vi "timestamp_to_postgres_date.vi"(8 "error in (no error)":errorcluster, 10 "utc":bool, 11 "date_time":dbl format="%^<%H:%M:%S%4u %m/%d/%y>T") -> (0 "error out":errorcluster, 3 "postgres_date":string)   [LabVIEW 2015, in "lv-example-postgres.lvlib"]
uses:
  lv-example-postgres.lvlib
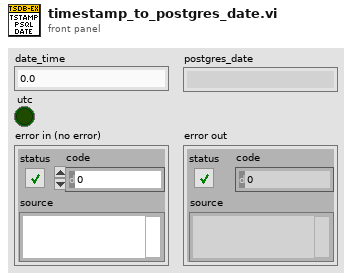
[diagram p1: front panel]
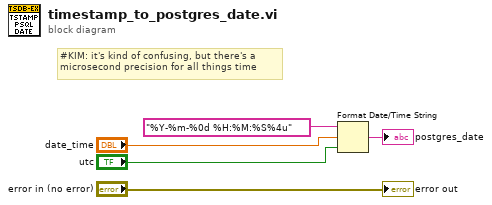
[diagram p0: block diagram]
diagram:
  # "#KIM: it's kind of confusing, but there's a \nmicrosecond precision for all things time"
  n1 = Format Date/Time String(time format string (%c)="%Y-%m-%0d %H:%M:%S%4u", seconds (now)="date_time", UTC format="utc") -> (date/time string=→"postgres_date":string)
  "error out" <- "error in (no error)"
